vi "Keysight XSAn - Example1.vi"() -> ()   [LabVIEW 2017]
doc: "This example initializes the driver, reads a few identity interface properties, and shows a few measurements."
uses:
  <instrlib>/Keysight XSAn/Keysight XSAn.lvlib
panel:
  out "Display Details":string
  in  "DEMO POWER SUITE MEASUREMENT":T1={"Center Frequency"=50000000.0, "Input Amplitude Reference"=0, "Frequency Span"=50000000.0, "Continuous MM"=TRUE, "Scale"=10.0} {"Frequency Span" format="%#.6f"; "Center Frequency" format="%#.6f"}
  in  "DEMO TRACE DATA READ":T1={"Center Frequency"=50000000.0, "Input Amplitude Reference"=0, "Frequency Span"=50000000.0, "Continuous MM"=TRUE, "Scale"=10.0} {"Frequency Span" format="%#.6f"; "Center Frequency" format="%#.6f"}
  in  "DEMO MARKER MEASUREMENT":T2={"Center Frequency"=50000000.0, "Input Amplitude Reference"=0, "Frequency Span"=50000000.0, "Continuous MM"=TRUE} {"Frequency Span" format="%#.6f"; "Center Frequency" format="%#.6f"}
  out "RetVal":dbl[](array[numeric]) caption="Power Suit Data" format="%.2p"
  out "RetValActualSize":i32 caption="Actual Size"
  in  "RetValBufferSize":i32=100 caption="Length"
  in  "MaxTime":i32=40000 caption="Maximum Time (ms)"
  in  "RepCapIdentifier":string="PST_Results" caption="RepCapIdentifier (PST_Results)"
  out "actual points":i32 caption="Actual Points"
  out "tracedata":dbl[](array[numeric]) caption="Trace Data"
  in  "array length":i32=10 caption="Array Length"
  in  "maximum time":i32=10000 caption="Maximum Time (ms)"
  in  "trace name":string="Trace1" caption="Trace Name (Trace1)"
  in  "Trigger Source":i32=3
  in  "Span 3":dbl=-90.0 caption="Peak Threshold (dB)" format="%#.6f"
  out "Marker Amplitude":dbl caption="Marker Amplitude (dB)"
  in  "marker search (Highest)":i32(ring)=1 items=["Highest"=1, "Minimum"=2, "Next Peak"=3, "Next Peak Left"=4, "Next Peak Right"=5]
  out "Marker Frequency":dbl caption="Marker Frequency (Hz)"
  out "Simulate":bool
  out "Info":T3
  in  "Simulate":bool=TRUE
  in  "Select ?":bool=TRUE
  in  "Resource String":string="PXI0::17-0.0::INSTR"
  in  "Options String":string="DriverSetup= Model=, Trace=false, TraceName=c:\\\\temp\\\\traceOut"
  # "Keysight XSAn - Example1"
  # "------------------------------------------------------------------------------------------------------------------------------------------------------------------------------------------------------------------------"
  # "------------------------------------------------------------------------------------------------------------------------------------------------------------------------------------------------------------------------------"
  # "© Keysight Technologies  2015-2018"
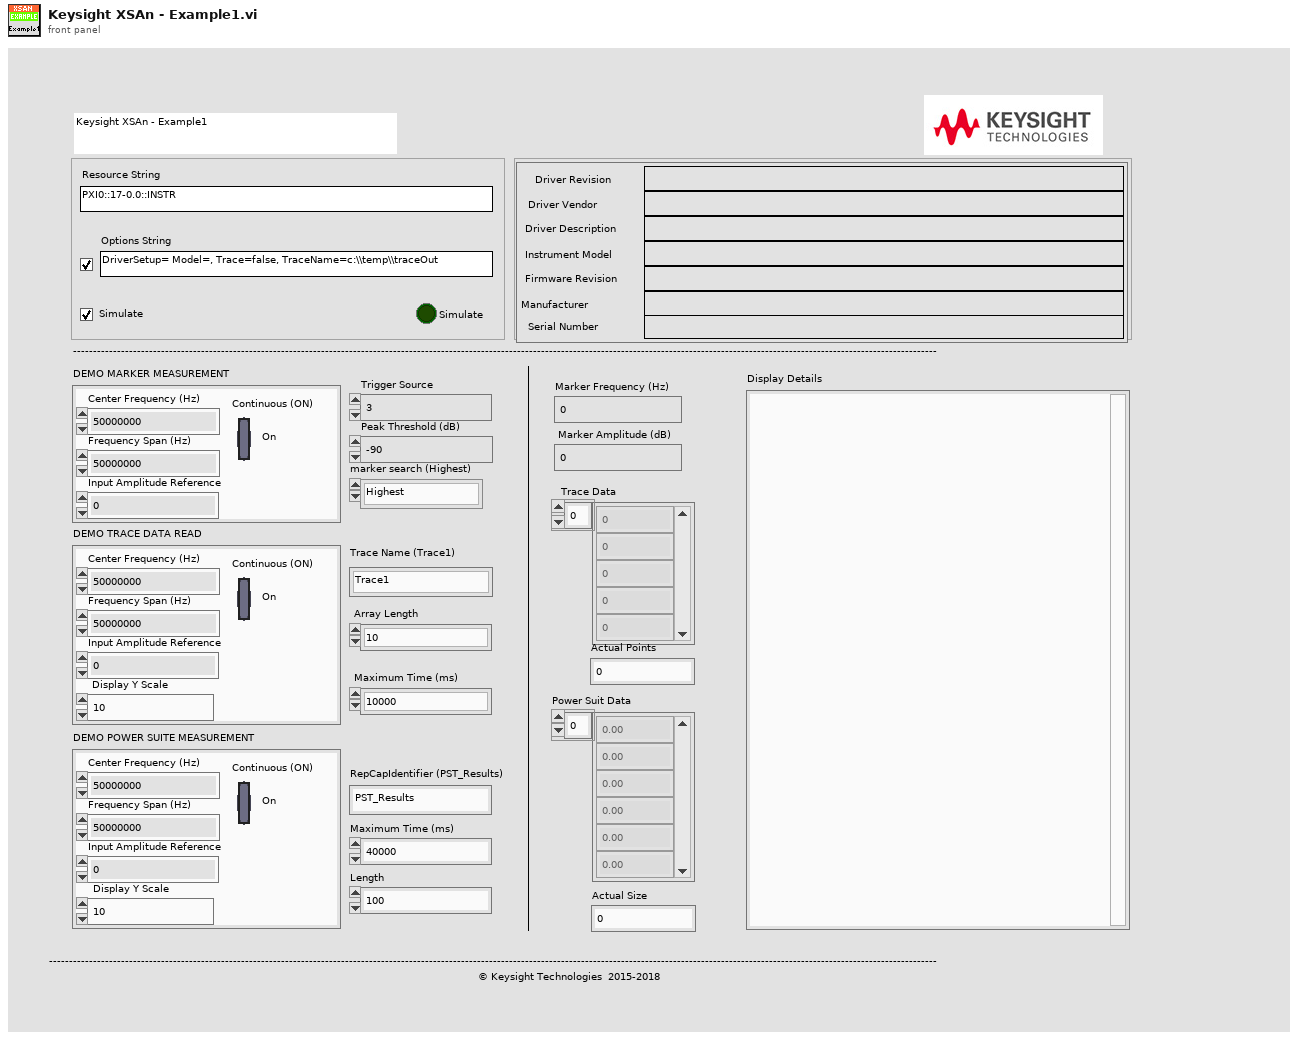
[diagram p1: front panel]
types:
  T1 = cluster{"Center Frequency":dbl, "Input Amplitude Reference":i32, "Frequency Span":dbl, "Continuous MM":bool, "Scale":dbl}
  T2 = cluster{"Center Frequency":dbl, "Input Amplitude Reference":i32, "Frequency Span":dbl, "Continuous MM":bool}
  T3 = cluster{"Driver Revision":string, "Driver Vendor":string, "Driver Description":string, "Instrument Model":string, "Firmware Revision":string, "Instrument Model 2":string, "Firmware Revision 2":string}
  T4 = cluster{"[0]":string, "[1]":string, "[2]":string, "[3]":string, "[4]":string, "[5]":string, "[6]":string}
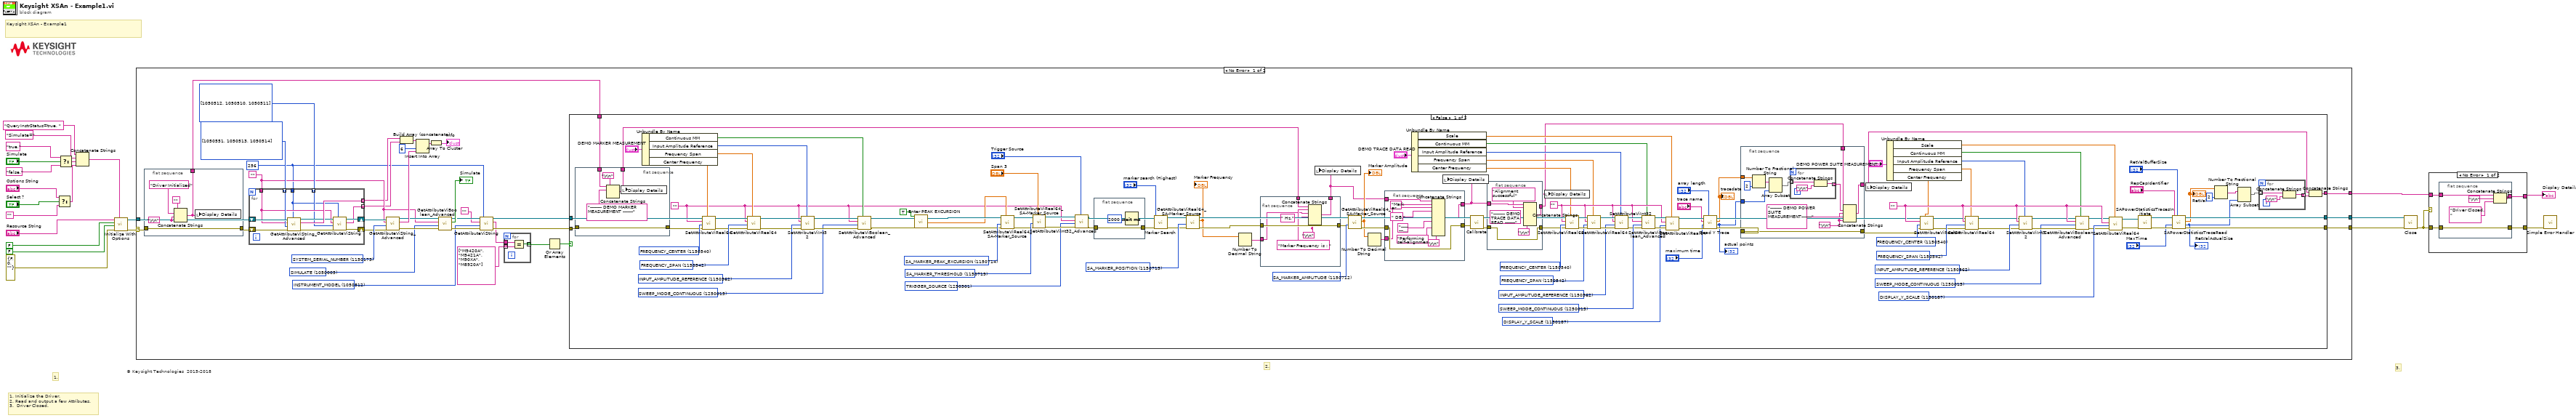
[diagram p0: block diagram]
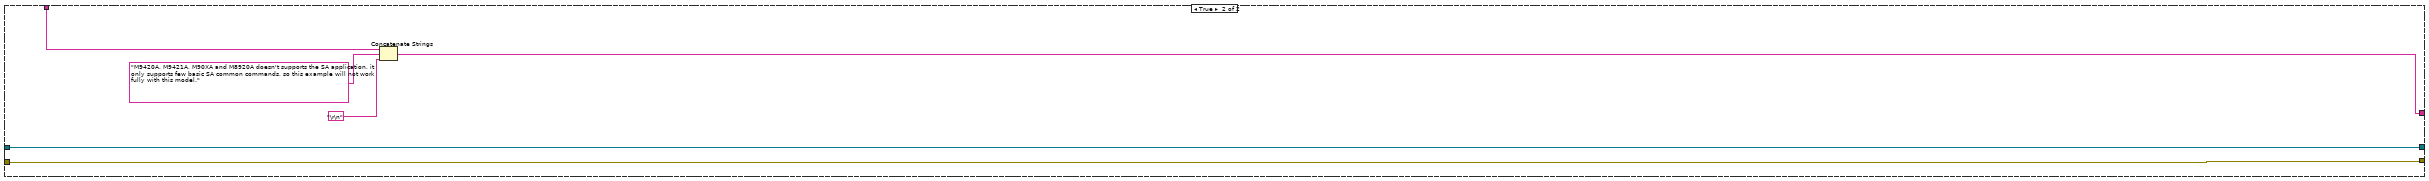
[diagram p3: hidden frame]
diagram:
  # "3."
  # "2."
  # "1."
  # "1. Initialize the Driver.\n2. Read and output a few Attributes.\n3.  Driver Closed."
  # "© Keysight Technologies  2015-2018"
  # "Keysight XSAn - Example1"
  n1 = Select(t="Options String", s="Select ?", f="") -> (s? t:f=w20:string)
  n2 = Select(t="true,", s="Simulate", f="false,") -> (s? t:f=w22:string)
  n3 = Concatenate Strings("QueryInstrStatus=true, " ("string"), "Simulate=" ("string"), w22, w20) -> (w12:string)
  n4 = call <instrlib>:"Initialize With Options.vi"("option string"=w12, "error in (no error)"=errorcluster {"status"=FALSE, "code"=0, "source"=""}, "reset device (Off)"=FALSE, "id query (Off)"=FALSE, "resource string"="Resource String") -> ("error out"=w13:errorcluster, "instrument handle out"=w7:refnum<k15>)  [unwired: 5 in]
  n5 = case shown="No Error" w13 {
    selector: w13 -> [w39 w258]
    tunnel: [w44 w258] -> w8
    tunnel: w7 -> [w37 w257]
    tunnel: [w43 w257] -> w5
    tunnel: [w35 _] -> w3
    frame No Error {
      w29 = u32 1050512 items=["ACTIVE_MARKER"=1250201, "CATALOG_CURRENT_MEASUREMENT_NAME"=1150676, "CATALOG_CURRENT_PERSONALITY_NAME"=1150677, "DISPLAY_TEXT"=1150119, "DRIVER_SETUP"=1050007, "INPUT_RF_CORRECTION_COMMENT"=1150737, "INPUT_RF_CORRECTION_DESCRIPTION"=1150738, "INSTRUMENT_FIRMWARE_REVISION"=1050510, "INSTRUMENT_MANUFACTURER"=1050511, "INSTRUMENT_MODEL"=1050512, "IO_RESOURCE_DESCRIPTOR"=1050304] ("AttributeID")
      w47 = u32 1050005 items=["IVILXISYNC_ARM_ALARM_ENABLED"=1950002, "IVILXISYNC_ARM_SOURCE_ENABLED"=1950011, "IVILXISYNC_ARM_SOURCE_OR_ENABLED"=1950014, "IVILXISYNC_EVENT_LOG_ENABLED"=1950034, "IVILXISYNC_IS_TIME_MASTER"=1950036, "IVILXISYNC_IS_TIME_SYNCHRONIZED"=1950037, "IVILXISYNC_TRIGGER_ALARM_ENABLED"=1950016, "LEVEL_ELECTRONIC_ATTENUATION_ENABLED"=1150583, "MARKER_ENABLED"=1250204, "MARKER_FREQUENCY_COUNTER_ENABLED"=1250205, "OUTPUT_ANALOG_AUTO_TYPE_ENABLED"=1150680, "PRESELECTOR_MW_ENABLED"=1150586, "RESOLUTION_BANDWIDTH_AUTO"=1250014, "SIGNAL_TRACK_ENABLED"=1250211, "SIMULATE"=1050005, "STATETRIGGER_ENABLED"=1150160, "SWEEP_MODE_CONTINUOUS"=1250015, "SWEEP_TIME_AUTO"=1250017, "SWEEP_TIME_ENABLED"=1150747, "SYSTEM_TRACE_ENABLED"=1150176, "TRACE_DISPLAY_ENABLED"=1150758, "TRACE_UPDATE_ENABLED"=1150757, "TRACES_AVERAGE_ENABLED"=1150756, "TRACES_AVERAGE_TYPE_AUTO_ENABLED"=1150667, "VIDEO_BANDWIDTH_AUTO"=1250023] ("AttributeID")
      w54 = u32 1150173 items=["IVILXISYNC_ARM_SOURCE_EVENTID"=1950012, "IVILXISYNC_ARM_SOURCE_FILTER"=1950013, "IVILXISYNC_EVENT_DESTINATION_PATH"=1950029, "IVILXISYNC_EVENT_SOURCE"=1950032, "IVILXISYNC_TRIGGER_SOURCE"=1950022, "IVILXISYNC_TRIGGER_SOURCE_EVENTID"=1950026, "IVILXISYNC_TRIGGER_SOURCE_FILTER"=1950027, "LOGICAL_NAME"=1050305, "MARKER_TRACE"=1250209, "SPECIFIC_DRIVER_DESCRIPTION"=1050514, "SPECIFIC_DRIVER_REVISION"=1050551, "SPECIFIC_DRIVER_VENDOR"=1050513, "STATETRIGGER_EVENT_ID"=1150161, "STATETRIGGER_FILTER"=1150162, "STATETRIGGER_STATE_LOCATION"=1150163, "SUPPORTED_INSTRUMENT_MODELS"=1050327, "SYSTEM_DATE"=1150172, "SYSTEM_SERIAL_NUMBER"=1150173, "SYSTEM_TIME"=1150174, "TEXT"=1150431] ("AttributeID")
      w57 = u32[] [1050512, 1050510, 1050511] items=["ACTIVE_MARKER"=1250201, "CATALOG_CURRENT_MEASUREMENT_NAME"=1150676, "CATALOG_CURRENT_PERSONALITY_NAME"=1150677, "DISPLAY_TEXT"=1150119, "DRIVER_SETUP"=1050007, "INPUT_RF_CORRECTION_COMMENT"=1150737, "INPUT_RF_CORRECTION_DESCRIPTION"=1150738, "INSTRUMENT_FIRMWARE_REVISION"=1050510, "INSTRUMENT_MANUFACTURER"=1050511, "INSTRUMENT_MODEL"=1050512, "IO_RESOURCE_DESCRIPTOR"=1050304]
      w46 = ""
      w28 = 256 ("AttributeValueBufferSize")
      w58 = u32[] [1050551, 1050513, 1050514] items=["IVILXISYNC_ARM_SOURCE_EVENTID"=1950012, "IVILXISYNC_ARM_SOURCE_FILTER"=1950013, "IVILXISYNC_EVENT_DESTINATION_PATH"=1950029, "IVILXISYNC_EVENT_SOURCE"=1950032, "IVILXISYNC_TRIGGER_SOURCE"=1950022, "IVILXISYNC_TRIGGER_SOURCE_EVENTID"=1950026, "IVILXISYNC_TRIGGER_SOURCE_FILTER"=1950027, "LOGICAL_NAME"=1050305, "MARKER_TRACE"=1250209, "SPECIFIC_DRIVER_DESCRIPTION"=1050514, "SPECIFIC_DRIVER_REVISION"=1050551, "SPECIFIC_DRIVER_VENDOR"=1050513, "STATETRIGGER_EVENT_ID"=1150161, "STATETRIGGER_FILTER"=1150162, "STATETRIGGER_STATE_LOCATION"=1150163, "SUPPORTED_INSTRUMENT_MODELS"=1050327, "SYSTEM_DATE"=1150172, "SYSTEM_SERIAL_NUMBER"=1150173, "SYSTEM_TIME"=1150174, "TEXT"=1150431]
      n6 = flat-sequence {
        tunnel: w39 -> [w66]
        tunnel: [w66] -> w38
        tunnel: [w63] -> w36
        frame #0 {
          w62 = "\r\n"
          n7 = Concatenate Strings("", "Driver Initialized", w62, w62) -> (w63:string)
          n8 = local write "Display Details"(w63) -> ()
        }
      }
      n9 = for {
        tunnel: w58 -> [w253] mode=indexing
        tunnel: [w254] -> w42 mode=indexing
        tunnel: w28 -> [w246]
        shift-right: [w250] -> w53
        shift-left: w37 -> [w256]
        shift-right: [w251] -> w52
        shift-left: w38 -> [w255]
        tunnel: w46 -> [w248]
        tunnel: w57 -> [w247] mode=indexing
        tunnel: [w245] -> w41 mode=indexing
        n10 = call <instrlib>:"GetAttributeViString_Advanced.vi"("AttributeValueBufferSize"=w246, "error in (no error)"=w255, "AttributeID"=w253, "RepCapIdentifier"=w248, "instrument handle"=w256) -> ("error out"=w252:errorcluster, "AttributeValue"=w254:string, "instrument handle out"=w249:refnum<k15>)  [unwired: 4 in]
        n11 = call <instrlib>:"GetAttributeViString.vi"("AttributeValueBufferSize"=w246, "error in (no error)"=w252, "AttributeID"=w247, "RepCapIdentifier"=w248, "instrument handle"=w249) -> ("error out"=w251:errorcluster, "AttributeValue"=w245:string, "instrument handle out"=w250:refnum<k15>)  [unwired: 4 in]
      }
      n12 = call <instrlib>:"GetAttributeViString_Advanced.vi"("error in (no error)"=w52, "AttributeID"=w54, "RepCapIdentifier"=w46, "instrument handle"=w53) -> ("error out"=w48:errorcluster, "AttributeValue"=w51:string, "instrument handle out"=w49:refnum<k15>)  [unwired: 5 in]
      n13 = Build Array (concatenate)(w42, w41) -> (w40:string[])
      n14 = Insert Into Array(array=w40, index=6, new element=w51) -> (w50:string[])
      n15 = Array To Cluster(array=w50) -> (cluster=→"Info":T4)
      n16 = call <instrlib>:"GetAttributeViBoolean_Advanced.vi"("error in (no error)"=w48, "AttributeID"=w47, "RepCapIdentifier"=w46, "instrument handle"=w49) -> ("error out"=w33:errorcluster, "AttributeValue"=→"Simulate":bool, "instrument handle out"=w34:refnum<k15>)  [unwired: 5 in]
      n17 = call <instrlib>:"GetAttributeViString.vi"("AttributeValueBufferSize"=w28, "error in (no error)"=w33, "AttributeID"=w29, "RepCapIdentifier"="", "instrument handle"=w34) -> ("error out"=w31:errorcluster, "AttributeValue"=w27:string, "instrument handle out"=w32:refnum<k15>)  [unwired: 4 in]
      n18 = for {
        tunnel: w27 -> [w61]
        tunnel: [w60] -> w25 mode=indexing
        tunnel: string[] ["M9420A", "M9421A", "M90XA", "M8920A"] -> [w59] mode=indexing
        n19 = Equal?(x=w61, y=w59) -> (x = y?=w60:bool)
      }
      n20 = Or Array Elements(Boolean array=w25) -> (logical OR=w24:bool)
      n21 = case shown="False" w24 {
        tunnel: w32 -> [w185 w244]
        tunnel: [w123 w243] -> w44
        tunnel: [w119 w244] -> w43
        tunnel: w31 -> [w97 w243]
        tunnel: w36 -> [w95 w241]
        tunnel: [w71 w239] -> w35
        frame False {
          w140 = u32 1150187 items=["ANALOGDEMODULATOR_CHANNEL_BANDWIDTH"=1150557, "ANALOGDEMODULATOR_TIME"=1150559, "ATTENUATION"=1250002, "DISPLAY_LINE"=1150191, "DISPLAY_NORMALIZED_REFERENCE"=1150184, "DISPLAY_REFERENCE_OFFSET"=1150186, "DISPLAY_REFERENCE"=1150185, "DISPLAY_Y_SCALE"=1150187, "EXTERNAL_MIXER_AVERAGE_CONVERSION_LOSS"=1250901, "EXTERNAL_MIXER_BIAS_LIMIT"=1250904, "EXTERNAL_MIXER_BIAS"=1250902, "EXTERNAL_TRIGGER_LEVEL"=1250401, "FREQUENCY_CENTER_STEP_INCREMENT"=1150541, "FREQUENCY_CENTER"=1150540, "FREQUENCY_OFFSET"=1250008, "FREQUENCY_SPAN_TO_RESOLUTION_BANDWIDTH_RATIO"=1150552, "FREQUENCY_SPAN"=1150542, "FREQUENCY_START"=1250006, "FREQUENCY_STOP"=1250007, "INPUT_IMPEDANCE"=1250009, "INPUT_RF_CENTER_FREQUENCY"=1150744, "INPUT_RF_CORRECTIONS_BASE_STATION_GAIN"=1150673, "INPUT_RF_CORRECTIONS_EXTERNAL_GAIN"=1150570, "INPUT_RF_CORRECTIONS_MOBILE_STATION_GAIN"=1150740, "INPUT_RF_MAX_MIXER_LEVEL"=1150572] ("AttributeID")
          w128 = u32 1250015 items=["IVILXISYNC_ARM_ALARM_ENABLED"=1950002, "IVILXISYNC_ARM_SOURCE_ENABLED"=1950011, "IVILXISYNC_ARM_SOURCE_OR_ENABLED"=1950014, "IVILXISYNC_EVENT_LOG_ENABLED"=1950034, "IVILXISYNC_TRIGGER_ALARM_ENABLED"=1950016, "LEVEL_ELECTRONIC_ATTENUATION_ENABLED"=1150583, "MARKER_ENABLED"=1250204, "MARKER_FREQUENCY_COUNTER_ENABLED"=1250205, "OUTPUT_ANALOG_AUTO_TYPE_ENABLED"=1150680, "PRESELECTOR_MW_ENABLED"=1150586, "RESOLUTION_BANDWIDTH_AUTO"=1250014, "SIGNAL_TRACK_ENABLED"=1250211, "SIMULATE"=1050005, "STATETRIGGER_ENABLED"=1150160, "SWEEP_MODE_CONTINUOUS"=1250015, "SWEEP_TIME_AUTO"=1250017, "SWEEP_TIME_ENABLED"=1150747, "SYSTEM_TRACE_ENABLED"=1150176, "TRACE_DISPLAY_ENABLED"=1150758, "TRACE_UPDATE_ENABLED"=1150757, "TRACES_AVERAGE_ENABLED"=1150756, "TRACES_AVERAGE_TYPE_AUTO_ENABLED"=1150667, "VIDEO_BANDWIDTH_AUTO"=1250023] ("AttributeID")
          w134 = u32 1150542 items=["ANALOGDEMODULATOR_CHANNEL_BANDWIDTH"=1150557, "ANALOGDEMODULATOR_TIME"=1150559, "ATTENUATION"=1250002, "DISPLAY_LINE"=1150191, "DISPLAY_NORMALIZED_REFERENCE"=1150184, "DISPLAY_REFERENCE_OFFSET"=1150186, "DISPLAY_REFERENCE"=1150185, "DISPLAY_Y_SCALE"=1150187, "EXTERNAL_MIXER_AVERAGE_CONVERSION_LOSS"=1250901, "EXTERNAL_MIXER_BIAS_LIMIT"=1250904, "EXTERNAL_MIXER_BIAS"=1250902, "EXTERNAL_TRIGGER_LEVEL"=1250401, "FREQUENCY_CENTER_STEP_INCREMENT"=1150541, "FREQUENCY_CENTER"=1150540, "FREQUENCY_OFFSET"=1250008, "FREQUENCY_SPAN_TO_RESOLUTION_BANDWIDTH_RATIO"=1150552, "FREQUENCY_SPAN"=1150542, "FREQUENCY_START"=1250006, "FREQUENCY_STOP"=1250007, "INPUT_IMPEDANCE"=1250009, "INPUT_RF_CENTER_FREQUENCY"=1150744, "INPUT_RF_CORRECTIONS_BASE_STATION_GAIN"=1150673, "INPUT_RF_CORRECTIONS_EXTERNAL_GAIN"=1150570, "INPUT_RF_CORRECTIONS_MOBILE_STATION_GAIN"=1150740, "INPUT_RF_MAX_MIXER_LEVEL"=1150572] ("AttributeID")
          w137 = u32 1150562 items=["AMPLITUDE_UNITS"=1250001, "ANALOGDEMODULATOR_FM_DE_EMPHASIS"=1150560, "ANALOGDEMODULATOR_TYPE"=1150556, "CALIBRATION_AUTO_ALERT_MODE"=1150674, "CALIBRATION_AUTO_ENABLED"=1150675, "DETECTOR_TYPE"=1250004, "DISPLAY_NORMALIZED_POSITION"=1150188, "DISPLAY_OPERATION_PRIORITY"=1150742, "DISPLAY_THEME"=1150155, "DISPLAY_VIEW"=1150743, "DISPLAY_WINDOW"=1150181, "EXTERNAL_MIXER_HARMONIC"=1250907, "EXTERNAL_MIXER_NUMBER_OF_PORTS"=1250908, "EXTERNAL_TRIGGER_SLOPE"=1250402, "FREQUENCY_SYNTHESIS"=1150543, "INPUT_AMPLITUDE_REFERENCE"=1150562, "INPUT_IF_FFT_IF_GAIN_STATE"=1150565, "INPUT_IF_SWEPT_IF_GAIN_STATE"=1150568, "INPUT_PORT"=1150563, "INPUT_RF_CORRECTION_ANTENNA_UNIT"=1150736, "INPUT_RF_CORRECTION_FREQUENCY_INTERPOLATION"=1150575, "INPUT_RF_CORRECTIONS_IMPEDANCE"=1150739, "INPUT_RF_COUPLING"=1150571, "INPUT_TYPE"=1150774] ("AttributeID")
          w141 = ""
          w136 = u32 1150540 items=["ANALOGDEMODULATOR_CHANNEL_BANDWIDTH"=1150557, "ANALOGDEMODULATOR_TIME"=1150559, "ATTENUATION"=1250002, "DISPLAY_LINE"=1150191, "DISPLAY_NORMALIZED_REFERENCE"=1150184, "DISPLAY_REFERENCE_OFFSET"=1150186, "DISPLAY_REFERENCE"=1150185, "DISPLAY_Y_SCALE"=1150187, "EXTERNAL_MIXER_AVERAGE_CONVERSION_LOSS"=1250901, "EXTERNAL_MIXER_BIAS_LIMIT"=1250904, "EXTERNAL_MIXER_BIAS"=1250902, "EXTERNAL_TRIGGER_LEVEL"=1250401, "FREQUENCY_CENTER_STEP_INCREMENT"=1150541, "FREQUENCY_CENTER"=1150540, "FREQUENCY_OFFSET"=1250008, "FREQUENCY_SPAN_TO_RESOLUTION_BANDWIDTH_RATIO"=1150552, "FREQUENCY_SPAN"=1150542, "FREQUENCY_START"=1250006, "FREQUENCY_STOP"=1250007, "INPUT_IMPEDANCE"=1250009, "INPUT_RF_CENTER_FREQUENCY"=1150744, "INPUT_RF_CORRECTIONS_BASE_STATION_GAIN"=1150673, "INPUT_RF_CORRECTIONS_EXTERNAL_GAIN"=1150570, "INPUT_RF_CORRECTIONS_MOBILE_STATION_GAIN"=1150740, "INPUT_RF_MAX_MIXER_LEVEL"=1150572] ("AttributeID")
          w148 = u32 1250301 items=["IVILXISYNC_ARM_ALARM_COUNT"=1950001, "IVILXISYNC_ARM_ALARM_REPEAT_COUNT"=1950004, "IVILXISYNC_ARM_COUNT"=1950007, "IVILXISYNC_ARM_SOURCE_COUNT"=1950009, "IVILXISYNC_ARM_SOURCE_DETECTION"=1950010, "IVILXISYNC_EVENT_COUNT"=1950028, "IVILXISYNC_EVENT_DRIVE_MODE"=1950030, "IVILXISYNC_EVENT_LOG_ENTRY_COUNT"=1950035, "IVILXISYNC_EVENT_SLOPE"=1950031, "IVILXISYNC_EVENT_WIRED_OR_BIAS_MODE"=1950033, "IVILXISYNC_TRIGGER_ALARM_COUNT"=1950015, "IVILXISYNC_TRIGGER_ALARM_REPEAT_COUNT"=1950018, "IVILXISYNC_TRIGGER_COUNT"=1950021, "IVILXISYNC_TRIGGER_SOURCE_COUNT"=1950023, "IVILXISYNC_TRIGGER_SOURCE_DETECTION"=1950025, "LEVEL_ATTENUATION_OPTIMIZE"=1150012, "LEVEL_ATTENUATION_STEP_INCREMENT"=1150013, "LEVEL_ELECTRONIC_ATTENUATION"=1150578, "MARKER_COUNT"=1250203, "MARKER_TYPE"=1250701, "MEMORYOPERATION_SCREEN_IMAGE_THEME"=1150678, "NUMBER_OF_DIVISIONS"=1250602, "NUMBER_OF_SWEEPS"=1250010, "OUTPUT_ANALOG_TYPE"=1150679, "OUTPUT_AUXILIARY_IF_TYPE"=1150681, "PRESELECTOR_MW_PATH"=1150585, "RADIO_BAND_CLASS"=1150550, "RADIO_DEVICE"=1150547, "RADIO_NON_STANDARD_MEASUREMENT_ENABLED"=1150549, "RADIO_PACKET_TYPE"=1150551, "RADIO_STANDARD"=1150548, "REFOSCILLATOR_EXTERNAL_BANDWIDTH"=1150539, "REFOSCILLATOR_EXTERNAL_COUPLING"=1150538, "STATETRIGGER_DETECTION"=1150159, "STATUS_SERIAL_POLL"=1150759, "SYSTEM_IO_TIMEOUT"=1150783, "SYSTEM_TIMEOUT_MILLISECONDS"=1150175, "TRACE_COUNT"=1250018, "TRACE_DETECTOR_TYPE"=1150782, "TRACE_SIZE"=1250019, "TRACE_TYPE"=1250020, "TRACES_AVERAGE_TYPE"=1150666, "TRIGGER_EXTERNAL2_SLOPE"=1150671, "TRIGGER_SOURCE"=1250301, "VERTICAL_SCALE"=1250021, "VIDEO_TRIGGER_SLOPE"=1250502] ("AttributeID")
          w156 = u32 1150719 items=["SA_MARKER_FREQUENCYCOUNTER_GATE_TIME"=1150683, "SA_MARKER_FUNCTION_BAND_LEFT"=1150693, "SA_MARKER_FUNCTION_BAND_RIGHT"=1150694, "SA_MARKER_FUNCTION_BAND_SPAN"=1150695, "SA_MARKER_NDBPOINTS_VALUE"=1150687, "SA_MARKER_PEAK_EXCURSION"=1150714, "SA_MARKER_POSITION"=1150715, "SA_MARKER_THRESHOLD"=1150719, "SA_MARKER_X_AXIS_TRACE_POINTS"=1150710, "SA_MARKER_Y"=1150702, "SA_SOURCE_FREQUENCY_OFFSET"=1150797, "SA_SOURCE_LEVEL_AMPLITUDE"=1150785, "SA_SOURCE_LEVEL_AMPLITUDE_OFFSET"=1150790, "SA_SOURCE_LEVEL_AMPLITUDE_STEP"=1150791, "SA_SOURCE_LEVEL_POWER_SWEEP"=1150788, "SA_SOURCE_LEVEL_TRACK_DELAY"=1150793] ("AttributeID")
          w157 = u32 1150714 items=["SA_MARKER_FREQUENCYCOUNTER_GATE_TIME"=1150683, "SA_MARKER_FUNCTION_BAND_LEFT"=1150693, "SA_MARKER_FUNCTION_BAND_RIGHT"=1150694, "SA_MARKER_FUNCTION_BAND_SPAN"=1150695, "SA_MARKER_NDBPOINTS_VALUE"=1150687, "SA_MARKER_PEAK_EXCURSION"=1150714, "SA_MARKER_POSITION"=1150715, "SA_MARKER_THRESHOLD"=1150719, "SA_MARKER_X_AXIS_TRACE_POINTS"=1150710, "SA_MARKER_Y"=1150702, "SA_SOURCE_FREQUENCY_OFFSET"=1150797, "SA_SOURCE_LEVEL_AMPLITUDE"=1150785, "SA_SOURCE_LEVEL_AMPLITUDE_OFFSET"=1150790, "SA_SOURCE_LEVEL_AMPLITUDE_STEP"=1150791, "SA_SOURCE_LEVEL_POWER_SWEEP"=1150788, "SA_SOURCE_LEVEL_TRACK_DELAY"=1150793] ("AttributeID")
          w160 = u32 1150187 items=["ANALOGDEMODULATOR_CHANNEL_BANDWIDTH"=1150557, "ANALOGDEMODULATOR_TIME"=1150559, "ATTENUATION"=1250002, "DISPLAY_LINE"=1150191, "DISPLAY_NORMALIZED_REFERENCE"=1150184, "DISPLAY_REFERENCE_OFFSET"=1150186, "DISPLAY_REFERENCE"=1150185, "DISPLAY_Y_SCALE"=1150187, "EXTERNAL_MIXER_AVERAGE_CONVERSION_LOSS"=1250901, "EXTERNAL_MIXER_BIAS_LIMIT"=1250904, "EXTERNAL_MIXER_BIAS"=1250902, "EXTERNAL_TRIGGER_LEVEL"=1250401, "FREQUENCY_CENTER_STEP_INCREMENT"=1150541, "FREQUENCY_CENTER"=1150540, "FREQUENCY_OFFSET"=1250008, "FREQUENCY_SPAN_TO_RESOLUTION_BANDWIDTH_RATIO"=1150552, "FREQUENCY_SPAN"=1150542, "FREQUENCY_START"=1250006, "FREQUENCY_STOP"=1250007, "INPUT_IMPEDANCE"=1250009, "INPUT_RF_CENTER_FREQUENCY"=1150744, "INPUT_RF_CORRECTIONS_BASE_STATION_GAIN"=1150673, "INPUT_RF_CORRECTIONS_EXTERNAL_GAIN"=1150570, "INPUT_RF_CORRECTIONS_MOBILE_STATION_GAIN"=1150740, "INPUT_RF_MAX_MIXER_LEVEL"=1150572] ("AttributeID")
          w173 = u32 1250015 items=["IVILXISYNC_ARM_ALARM_ENABLED"=1950002, "IVILXISYNC_ARM_SOURCE_ENABLED"=1950011, "IVILXISYNC_ARM_SOURCE_OR_ENABLED"=1950014, "IVILXISYNC_EVENT_LOG_ENABLED"=1950034, "IVILXISYNC_TRIGGER_ALARM_ENABLED"=1950016, "LEVEL_ELECTRONIC_ATTENUATION_ENABLED"=1150583, "MARKER_ENABLED"=1250204, "MARKER_FREQUENCY_COUNTER_ENABLED"=1250205, "OUTPUT_ANALOG_AUTO_TYPE_ENABLED"=1150680, "PRESELECTOR_MW_ENABLED"=1150586, "RESOLUTION_BANDWIDTH_AUTO"=1250014, "SIGNAL_TRACK_ENABLED"=1250211, "SIMULATE"=1050005, "STATETRIGGER_ENABLED"=1150160, "SWEEP_MODE_CONTINUOUS"=1250015, "SWEEP_TIME_AUTO"=1250017, "SWEEP_TIME_ENABLED"=1150747, "SYSTEM_TRACE_ENABLED"=1150176, "TRACE_DISPLAY_ENABLED"=1150758, "TRACE_UPDATE_ENABLED"=1150757, "TRACES_AVERAGE_ENABLED"=1150756, "TRACES_AVERAGE_TYPE_AUTO_ENABLED"=1150667, "VIDEO_BANDWIDTH_AUTO"=1250023] ("AttributeID")
          w167 = u32 1150542 items=["ANALOGDEMODULATOR_CHANNEL_BANDWIDTH"=1150557, "ANALOGDEMODULATOR_TIME"=1150559, "ATTENUATION"=1250002, "DISPLAY_LINE"=1150191, "DISPLAY_NORMALIZED_REFERENCE"=1150184, "DISPLAY_REFERENCE_OFFSET"=1150186, "DISPLAY_REFERENCE"=1150185, "DISPLAY_Y_SCALE"=1150187, "EXTERNAL_MIXER_AVERAGE_CONVERSION_LOSS"=1250901, "EXTERNAL_MIXER_BIAS_LIMIT"=1250904, "EXTERNAL_MIXER_BIAS"=1250902, "EXTERNAL_TRIGGER_LEVEL"=1250401, "FREQUENCY_CENTER_STEP_INCREMENT"=1150541, "FREQUENCY_CENTER"=1150540, "FREQUENCY_OFFSET"=1250008, "FREQUENCY_SPAN_TO_RESOLUTION_BANDWIDTH_RATIO"=1150552, "FREQUENCY_SPAN"=1150542, "FREQUENCY_START"=1250006, "FREQUENCY_STOP"=1250007, "INPUT_IMPEDANCE"=1250009, "INPUT_RF_CENTER_FREQUENCY"=1150744, "INPUT_RF_CORRECTIONS_BASE_STATION_GAIN"=1150673, "INPUT_RF_CORRECTIONS_EXTERNAL_GAIN"=1150570, "INPUT_RF_CORRECTIONS_MOBILE_STATION_GAIN"=1150740, "INPUT_RF_MAX_MIXER_LEVEL"=1150572] ("AttributeID")
          w164 = u32 1150562 items=["AMPLITUDE_UNITS"=1250001, "ANALOGDEMODULATOR_FM_DE_EMPHASIS"=1150560, "ANALOGDEMODULATOR_TYPE"=1150556, "CALIBRATION_AUTO_ALERT_MODE"=1150674, "CALIBRATION_AUTO_ENABLED"=1150675, "DETECTOR_TYPE"=1250004, "DISPLAY_NORMALIZED_POSITION"=1150188, "DISPLAY_OPERATION_PRIORITY"=1150742, "DISPLAY_THEME"=1150155, "DISPLAY_VIEW"=1150743, "DISPLAY_WINDOW"=1150181, "EXTERNAL_MIXER_HARMONIC"=1250907, "EXTERNAL_MIXER_NUMBER_OF_PORTS"=1250908, "EXTERNAL_TRIGGER_SLOPE"=1250402, "FREQUENCY_SYNTHESIS"=1150543, "INPUT_AMPLITUDE_REFERENCE"=1150562, "INPUT_IF_FFT_IF_GAIN_STATE"=1150565, "INPUT_IF_SWEPT_IF_GAIN_STATE"=1150568, "INPUT_PORT"=1150563, "INPUT_RF_CORRECTION_ANTENNA_UNIT"=1150736, "INPUT_RF_CORRECTION_FREQUENCY_INTERPOLATION"=1150575, "INPUT_RF_CORRECTIONS_IMPEDANCE"=1150739, "INPUT_RF_COUPLING"=1150571, "INPUT_TYPE"=1150774] ("AttributeID")
          w159 = ""
          w165 = u32 1150540 items=["ANALOGDEMODULATOR_CHANNEL_BANDWIDTH"=1150557, "ANALOGDEMODULATOR_TIME"=1150559, "ATTENUATION"=1250002, "DISPLAY_LINE"=1150191, "DISPLAY_NORMALIZED_REFERENCE"=1150184, "DISPLAY_REFERENCE_OFFSET"=1150186, "DISPLAY_REFERENCE"=1150185, "DISPLAY_Y_SCALE"=1150187, "EXTERNAL_MIXER_AVERAGE_CONVERSION_LOSS"=1250901, "EXTERNAL_MIXER_BIAS_LIMIT"=1250904, "EXTERNAL_MIXER_BIAS"=1250902, "EXTERNAL_TRIGGER_LEVEL"=1250401, "FREQUENCY_CENTER_STEP_INCREMENT"=1150541, "FREQUENCY_CENTER"=1150540, "FREQUENCY_OFFSET"=1250008, "FREQUENCY_SPAN_TO_RESOLUTION_BANDWIDTH_RATIO"=1150552, "FREQUENCY_SPAN"=1150542, "FREQUENCY_START"=1250006, "FREQUENCY_STOP"=1250007, "INPUT_IMPEDANCE"=1250009, "INPUT_RF_CENTER_FREQUENCY"=1150744, "INPUT_RF_CORRECTIONS_BASE_STATION_GAIN"=1150673, "INPUT_RF_CORRECTIONS_EXTERNAL_GAIN"=1150570, "INPUT_RF_CORRECTIONS_MOBILE_STATION_GAIN"=1150740, "INPUT_RF_MAX_MIXER_LEVEL"=1150572] ("AttributeID")
          w174 = u32 1250015 items=["IVILXISYNC_ARM_ALARM_ENABLED"=1950002, "IVILXISYNC_ARM_SOURCE_ENABLED"=1950011, "IVILXISYNC_ARM_SOURCE_OR_ENABLED"=1950014, "IVILXISYNC_EVENT_LOG_ENABLED"=1950034, "IVILXISYNC_TRIGGER_ALARM_ENABLED"=1950016, "LEVEL_ELECTRONIC_ATTENUATION_ENABLED"=1150583, "MARKER_ENABLED"=1250204, "MARKER_FREQUENCY_COUNTER_ENABLED"=1250205, "OUTPUT_ANALOG_AUTO_TYPE_ENABLED"=1150680, "PRESELECTOR_MW_ENABLED"=1150586, "RESOLUTION_BANDWIDTH_AUTO"=1250014, "SIGNAL_TRACK_ENABLED"=1250211, "SIMULATE"=1050005, "STATETRIGGER_ENABLED"=1150160, "SWEEP_MODE_CONTINUOUS"=1250015, "SWEEP_TIME_AUTO"=1250017, "SWEEP_TIME_ENABLED"=1150747, "SYSTEM_TRACE_ENABLED"=1150176, "TRACE_DISPLAY_ENABLED"=1150758, "TRACE_UPDATE_ENABLED"=1150757, "TRACES_AVERAGE_ENABLED"=1150756, "TRACES_AVERAGE_TYPE_AUTO_ENABLED"=1150667, "VIDEO_BANDWIDTH_AUTO"=1250023] ("AttributeID")
          w182 = u32 1150715 items=["SA_MARKER_AMPLITUDE"=1150712, "SA_MARKER_FREQUENCYCOUNTER_GATE_TIME"=1150683, "SA_MARKER_FUNCTION_BAND_LEFT"=1150693, "SA_MARKER_FUNCTION_BAND_RIGHT"=1150694, "SA_MARKER_FUNCTION_BAND_SPAN"=1150695, "SA_MARKER_NDBPOINTS_RESULTS"=1150688, "SA_MARKER_NDBPOINTS_VALUE"=1150687, "SA_MARKER_PEAK_EXCURSION"=1150714, "SA_MARKER_POSITION"=1150715, "SA_MARKER_REFERENCE_AMPLITUDE"=1150716, "SA_MARKER_REFERENCE_POSITION"=1150717, "SA_MARKER_THRESHOLD"=1150719, "SA_MARKER_X_AXIS_TRACE_POINTS"=1150710, "SA_MARKER_Y"=1150702, "SA_SOURCE_FREQUENCY_OFFSET"=1150797, "SA_SOURCE_LEVEL_AMPLITUDE"=1150785, "SA_SOURCE_LEVEL_AMPLITUDE_OFFSET"=1150790, "SA_SOURCE_LEVEL_AMPLITUDE_STEP"=1150791, "SA_SOURCE_LEVEL_POWER_SWEEP"=1150788, "SA_SOURCE_LEVEL_TRACK_DELAY"=1150793] ("AttributeID")
          w181 = u32 1150712 items=["SA_MARKER_AMPLITUDE"=1150712, "SA_MARKER_FREQUENCYCOUNTER_GATE_TIME"=1150683, "SA_MARKER_FUNCTION_BAND_LEFT"=1150693, "SA_MARKER_FUNCTION_BAND_RIGHT"=1150694, "SA_MARKER_FUNCTION_BAND_SPAN"=1150695, "SA_MARKER_NDBPOINTS_RESULTS"=1150688, "SA_MARKER_NDBPOINTS_VALUE"=1150687, "SA_MARKER_PEAK_EXCURSION"=1150714, "SA_MARKER_POSITION"=1150715, "SA_MARKER_REFERENCE_AMPLITUDE"=1150716, "SA_MARKER_REFERENCE_POSITION"=1150717, "SA_MARKER_THRESHOLD"=1150719, "SA_MARKER_X_AXIS_TRACE_POINTS"=1150710, "SA_MARKER_Y"=1150702, "SA_SOURCE_FREQUENCY_OFFSET"=1150797, "SA_SOURCE_LEVEL_AMPLITUDE"=1150785, "SA_SOURCE_LEVEL_AMPLITUDE_OFFSET"=1150790, "SA_SOURCE_LEVEL_AMPLITUDE_STEP"=1150791, "SA_SOURCE_LEVEL_POWER_SWEEP"=1150788, "SA_SOURCE_LEVEL_TRACK_DELAY"=1150793] ("AttributeID")
          w189 = u32 1150542 items=["ANALOGDEMODULATOR_CHANNEL_BANDWIDTH"=1150557, "ANALOGDEMODULATOR_TIME"=1150559, "ATTENUATION"=1250002, "DISPLAY_LINE"=1150191, "DISPLAY_NORMALIZED_REFERENCE"=1150184, "DISPLAY_REFERENCE_OFFSET"=1150186, "DISPLAY_REFERENCE"=1150185, "DISPLAY_Y_SCALE"=1150187, "EXTERNAL_MIXER_AVERAGE_CONVERSION_LOSS"=1250901, "EXTERNAL_MIXER_BIAS_LIMIT"=1250904, "EXTERNAL_MIXER_BIAS"=1250902, "EXTERNAL_TRIGGER_LEVEL"=1250401, "FREQUENCY_CENTER_STEP_INCREMENT"=1150541, "FREQUENCY_CENTER"=1150540, "FREQUENCY_OFFSET"=1250008, "FREQUENCY_SPAN_TO_RESOLUTION_BANDWIDTH_RATIO"=1150552, "FREQUENCY_SPAN"=1150542, "FREQUENCY_START"=1250006, "FREQUENCY_STOP"=1250007, "INPUT_IMPEDANCE"=1250009, "INPUT_RF_CENTER_FREQUENCY"=1150744, "INPUT_RF_CORRECTIONS_BASE_STATION_GAIN"=1150673, "INPUT_RF_CORRECTIONS_EXTERNAL_GAIN"=1150570, "INPUT_RF_CORRECTIONS_MOBILE_STATION_GAIN"=1150740, "INPUT_RF_MAX_MIXER_LEVEL"=1150572] ("AttributeID")
          w192 = u32 1150562 items=["AMPLITUDE_UNITS"=1250001, "ANALOGDEMODULATOR_FM_DE_EMPHASIS"=1150560, "ANALOGDEMODULATOR_TYPE"=1150556, "CALIBRATION_AUTO_ALERT_MODE"=1150674, "CALIBRATION_AUTO_ENABLED"=1150675, "DETECTOR_TYPE"=1250004, "DISPLAY_NORMALIZED_POSITION"=1150188, "DISPLAY_OPERATION_PRIORITY"=1150742, "DISPLAY_THEME"=1150155, "DISPLAY_VIEW"=1150743, "DISPLAY_WINDOW"=1150181, "EXTERNAL_MIXER_HARMONIC"=1250907, "EXTERNAL_MIXER_NUMBER_OF_PORTS"=1250908, "EXTERNAL_TRIGGER_SLOPE"=1250402, "FREQUENCY_SYNTHESIS"=1150543, "INPUT_AMPLITUDE_REFERENCE"=1150562, "INPUT_IF_FFT_IF_GAIN_STATE"=1150565, "INPUT_IF_SWEPT_IF_GAIN_STATE"=1150568, "INPUT_PORT"=1150563, "INPUT_RF_CORRECTION_ANTENNA_UNIT"=1150736, "INPUT_RF_CORRECTION_FREQUENCY_INTERPOLATION"=1150575, "INPUT_RF_CORRECTIONS_IMPEDANCE"=1150739, "INPUT_RF_COUPLING"=1150571, "INPUT_TYPE"=1150774] ("AttributeID")
          w77 = ""
          w191 = u32 1150540 items=["ANALOGDEMODULATOR_CHANNEL_BANDWIDTH"=1150557, "ANALOGDEMODULATOR_TIME"=1150559, "ATTENUATION"=1250002, "DISPLAY_LINE"=1150191, "DISPLAY_NORMALIZED_REFERENCE"=1150184, "DISPLAY_REFERENCE_OFFSET"=1150186, "DISPLAY_REFERENCE"=1150185, "DISPLAY_Y_SCALE"=1150187, "EXTERNAL_MIXER_AVERAGE_CONVERSION_LOSS"=1250901, "EXTERNAL_MIXER_BIAS_LIMIT"=1250904, "EXTERNAL_MIXER_BIAS"=1250902, "EXTERNAL_TRIGGER_LEVEL"=1250401, "FREQUENCY_CENTER_STEP_INCREMENT"=1150541, "FREQUENCY_CENTER"=1150540, "FREQUENCY_OFFSET"=1250008, "FREQUENCY_SPAN_TO_RESOLUTION_BANDWIDTH_RATIO"=1150552, "FREQUENCY_SPAN"=1150542, "FREQUENCY_START"=1250006, "FREQUENCY_STOP"=1250007, "INPUT_IMPEDANCE"=1250009, "INPUT_RF_CENTER_FREQUENCY"=1150744, "INPUT_RF_CORRECTIONS_BASE_STATION_GAIN"=1150673, "INPUT_RF_CORRECTIONS_EXTERNAL_GAIN"=1150570, "INPUT_RF_CORRECTIONS_MOBILE_STATION_GAIN"=1150740, "INPUT_RF_MAX_MIXER_LEVEL"=1150572] ("AttributeID")
          n22 = flat-sequence {
            tunnel: w97 -> [w236]
            tunnel: [w236] -> w96
            tunnel: w95 -> [w235]
            tunnel: [w233] -> w92
            frame #0 {
              w232 = "\r\n"
              n23 = Concatenate Strings(w235, "-------- DEMO MARKER MEASUREMENT -------" ("y"), w232, w232) -> (w233:string)
              n24 = local write "Display Details"(w233) -> ()
            }
          }
          n25 = Unbundle By Name("DEMO MARKER MEASUREMENT") -> ("Continuous MM"=w113:bool, "Input Amplitude Reference"=w112:i32, "Frequency Span"=w111:dbl, "Center Frequency"=w110:dbl)
          n26 = call <instrlib>:"SetAttributeViReal64.vi"("AttributeValue"=w110, "error in (no error)"=w96, "AttributeID"=w191, "RepCapIdentifier"=w77, "instrument handle"=w185) -> ("error out"=w186:errorcluster, "instrument handle out"=w190:refnum<k15>)  [unwired: 5 in]
          n27 = call <instrlib>:"SetAttributeViReal64.vi"("AttributeValue"=w111, "error in (no error)"=w186, "AttributeID"=w189, "RepCapIdentifier"=w77, "instrument handle"=w190) -> ("error out"=w187:errorcluster, "instrument handle out"=w188:refnum<k15>)  [unwired: 5 in]
          n28 = call <instrlib>:"SetAttributeViInt32.vi"("AttributeValue"=w112, "error in (no error)"=w187, "AttributeID"=w192, "RepCapIdentifier"=w77, "instrument handle"=w188) -> ("error out"=w175:errorcluster, "instrument handle out"=w176:refnum<k15>)  [unwired: 5 in]
          n29 = call <instrlib>:"SetAttributeViBoolean_Advanced.vi"("AttributeValue (Off)"=w113, "error in (no error)"=w175, "AttributeID"=w174, "RepCapIdentifier"=w77, "instrument handle"=w176) -> ("error out"=w118:errorcluster, "instrument handle out"=w158:refnum<k15>)  [unwired: 5 in]
          n30 = call "Enter PEAK EXCURSION"("Enable"=TRUE, "error in (no error)"=w118) -> ("PEAK EXCURSION"=w116:dbl, "error out"=w117:errorcluster)  [unwired: 15 in, 1 out]
          n31 = call <instrlib>:"SetAttributeViReal64_SA-Marker_Source.vi"("AttributeValue"=w116, "error in (no error)"=w117, "AttributeID"=w157, "instrument handle"=w158) -> ("error out"=w154:errorcluster, "instrument handle out"=w155:refnum<k15>)  [unwired: 6 in]
          n32 = call <instrlib>:"SetAttributeViReal64_SA-Marker_Source.vi"("AttributeValue"="Span 3", "error in (no error)"=w154, "AttributeID"=w156, "instrument handle"=w155) -> ("error out"=w151:errorcluster, "instrument handle out"=w152:refnum<k15>)  [unwired: 6 in]
          n33 = call <instrlib>:"SetAttributeViInt32_Advanced.vi"("AttributeValue"="Trigger Source", "error in (no error)"=w151, "AttributeID"=w148, "RepCapIdentifier"=w77, "instrument handle"=w152) -> ("error out"=w149:errorcluster, "instrument handle out"=w150:refnum<k15>)  [unwired: 5 in]
          n34 = flat-sequence {
            tunnel: w149 -> [w237]
            tunnel: [w237] -> w184
            frame #0 {
              n35 = Wait (ms)(milliseconds to wait=u32 2000) -> ()  [unwired: 1 out]
            }
          }
          n36 = call <instrlib>:"Marker Search.vi"("error in (no error)"=w184, "marker search (Highest)"="marker search (Highest)", "instrument handle"=w150) -> ("error out"=w178:errorcluster, "instrument handle out"=w180:refnum<k15>)  [unwired: 7 in]
          n37 = call <instrlib>:"GetAttributeViReal64_SA-Marker_Source.vi"("error in (no error)"=w178, "AttributeID"=w182, "instrument handle"=w180) -> ("error out"=w94:errorcluster, "AttributeValue"=w91:dbl, "instrument handle out"=w179:refnum<k15>)  [unwired: 6 in]
          "Marker Frequency" <- w91
          n38 = Number To Decimal String(number=w91) -> (decimal integer string=w90:string)  [unwired: 1 in]
          n39 = flat-sequence {
            tunnel: w94 -> [w231]
            tunnel: [w231] -> w93
            tunnel: w92 -> [w230]
            tunnel: w90 -> [w228]
            tunnel: [w226] -> w85
            frame #0 {
              w225 = "\r\n"
              n40 = Concatenate Strings(w230, "Marker Frequency is : ", w228, " Hz.", w225, w225) -> (w226:string)
            }
          }
          n41 = local write "Display Details"(w85) -> ()
          n42 = call <instrlib>:"GetAttributeViReal64_SA-Marker_Source.vi"("error in (no error)"=w93, "AttributeID"=w181, "instrument handle"=w179) -> ("error out"=w89:errorcluster, "AttributeValue"=w87:dbl, "instrument handle out"=w177:refnum<k15>)  [unwired: 6 in]
          "Marker Amplitude" <- w87
          n43 = Number To Decimal String(number=w87) -> (decimal integer string=w86:string)  [unwired: 1 in]
          n44 = flat-sequence {
            tunnel: [w224] -> w83
            tunnel: w89 -> [w221]
            tunnel: [w221] -> w88
            tunnel: w86 -> [w220]
            tunnel: w85 -> [w219]
            frame #0 {
              w216 = "\r\n"
              n45 = Concatenate Strings(w219, "Marker Amplitude is : ", w220, " DB.", w216, w216, "-------- DEMO INTERNAL ALIGNMENT -------" ("y"), w216, "Performing self-alignment..." ("y"), w216, w216) -> (w224:string)
            }
          }
          n46 = Unbundle By Name("DEMO TRACE DATA READ") -> ("Scale"=w99:dbl, "Continuous MM"=w105:bool, "Input Amplitude Reference"=w106:i32, "Frequency Span"=w107:dbl, "Center Frequency"=w108:dbl)
          n47 = local write "Display Details"(w83) -> ()
          n48 = call <instrlib>:"Calibrate.vi"("error in (no error)"=w88, "instrument handle"=w177) -> ("error out"=w84:errorcluster, "instrument handle out"=w163:refnum<k15>)  [unwired: 8 in]
          n49 = flat-sequence {
            tunnel: w84 -> [w212]
            tunnel: w83 -> [w215]
            tunnel: [w213] -> w79
            tunnel: [w212] -> w82
            frame #0 {
              w210 = "\r\n"
              n50 = Concatenate Strings(w215, "Alignment successful" ("y"), w210, w210, "-------- DEMO TRACE DATA READ -------" ("y"), w210, w210) -> (w213:string)
            }
          }
          n51 = local write "Display Details"(w79) -> ()
          n52 = call <instrlib>:"SetAttributeViReal64.vi"("AttributeValue"=w108, "error in (no error)"=w82, "AttributeID"=w165, "RepCapIdentifier"=w159, "instrument handle"=w163) -> ("error out"=w170:errorcluster, "instrument handle out"=w166:refnum<k15>)  [unwired: 5 in]
          n53 = call <instrlib>:"SetAttributeViReal64.vi"("AttributeValue"=w107, "error in (no error)"=w170, "AttributeID"=w167, "RepCapIdentifier"=w159, "instrument handle"=w166) -> ("error out"=w169:errorcluster, "instrument handle out"=w168:refnum<k15>)  [unwired: 5 in]
          n54 = call <instrlib>:"SetAttributeViInt32.vi"("AttributeValue"=w106, "error in (no error)"=w169, "AttributeID"=w164, "RepCapIdentifier"=w159, "instrument handle"=w168) -> ("error out"=w172:errorcluster, "instrument handle out"=w171:refnum<k15>)  [unwired: 5 in]
          n55 = call <instrlib>:"SetAttributeViBoolean_Advanced.vi"("AttributeValue (Off)"=w105, "error in (no error)"=w172, "AttributeID"=w173, "RepCapIdentifier"=w159, "instrument handle"=w171) -> ("error out"=w161:errorcluster, "instrument handle out"=w162:refnum<k15>)  [unwired: 5 in]
          n56 = call <instrlib>:"SetAttributeViReal64.vi"("AttributeValue"=w99, "error in (no error)"=w161, "AttributeID"=w160, "RepCapIdentifier"=w159, "instrument handle"=w162) -> ("error out"=w145:errorcluster, "instrument handle out"=w146:refnum<k15>)  [unwired: 5 in]
          n57 = call <instrlib>:"Read Y Trace.vi"("array length"="array length", "error in (no error)"=w145, "maximum time"="maximum time", "trace name"="trace name", "instrument handle"=w146) -> ("error out"=w81:errorcluster, "actual points"=w70:i32, "amplitude"=w76:dbl[], "instrument handle out"=w127:refnum<k15>)  [unwired: 3 in]
          "tracedata" <- w76
          "actual points" <- w70
          n58 = flat-sequence {
            tunnel: w81 -> [w206]
            tunnel: [w206] -> w80
            tunnel: w79 -> [w205]
            tunnel: [w204] -> w73
            tunnel: w76 -> [w201]
            tunnel: w70 -> [w196]
            frame #0 {
              w202 = "\r\n"
              n59 = Number To Fractional String(number=w201, precision (6)=i16 2) -> (F-format string=w199:string[])  [unwired: 2 in]
              n60 = Array Subset(array=w199, length=w196) -> (w197:string[])  [unwired: 1 in]
              n61 = for {
                tunnel: w197 -> [w209] mode=indexing
                tunnel: [w207] -> w198 mode=indexing
                n62 = Concatenate Strings(w209, "\r\n") -> (w207:string)
              }
              n63 = Concatenate Strings(w205, w198, w202, "-------- DEMO POWER SUITE MEASUREMENT-------" ("y"), w202) -> (w204:string)
            }
          }
          n64 = local write "Display Details"(w73) -> ()
          n65 = Unbundle By Name("DEMO POWER SUITE MEASUREMENT") -> ("Scale"=w98:dbl, "Continuous MM"=w100:bool, "Input Amplitude Reference"=w101:i32, "Frequency Span"=w102:dbl, "Center Frequency"=w103:dbl)
          n66 = call <instrlib>:"SetAttributeViReal64.vi"("AttributeValue"=w103, "error in (no error)"=w80, "AttributeID"=w136, "RepCapIdentifier"=w141, "instrument handle"=w127) -> ("error out"=w131:errorcluster, "instrument handle out"=w135:refnum<k15>)  [unwired: 5 in]
          n67 = call <instrlib>:"SetAttributeViReal64.vi"("AttributeValue"=w102, "error in (no error)"=w131, "AttributeID"=w134, "RepCapIdentifier"=w141, "instrument handle"=w135) -> ("error out"=w132:errorcluster, "instrument handle out"=w133:refnum<k15>)  [unwired: 5 in]
          n68 = call <instrlib>:"SetAttributeViInt32.vi"("AttributeValue"=w101, "error in (no error)"=w132, "AttributeID"=w137, "RepCapIdentifier"=w141, "instrument handle"=w133) -> ("error out"=w129:errorcluster, "instrument handle out"=w130:refnum<k15>)  [unwired: 5 in]
          n69 = call <instrlib>:"SetAttributeViBoolean_Advanced.vi"("AttributeValue (Off)"=w100, "error in (no error)"=w129, "AttributeID"=w128, "RepCapIdentifier"=w141, "instrument handle"=w130) -> ("error out"=w139:errorcluster, "instrument handle out"=w138:refnum<k15>)  [unwired: 5 in]
          n70 = call <instrlib>:"SetAttributeViReal64.vi"("AttributeValue"=w98, "error in (no error)"=w139, "AttributeID"=w140, "RepCapIdentifier"=w141, "instrument handle"=w138) -> ("error out"=w78:errorcluster, "instrument handle out"=w126:refnum<k15>)  [unwired: 5 in]
          n71 = call <instrlib>:"SAPowerStatisticsTracesInitiate.vi"("error in (no error)"=w78, "instrument handle"=w126) -> ("error out"=w124:errorcluster, "instrument handle out"=w125:refnum<k15>)  [unwired: 8 in]
          n72 = call <instrlib>:"SAPowerStatisticsTraceRead.vi"("RetValBufferSize"="RetValBufferSize", "error in (no error)"=w124, "MaxTime"="MaxTime", "RepCapIdentifier"="RepCapIdentifier", "instrument handle"=w125) -> ("error out"=w123:errorcluster, "RetValActualSize"=w68:i32, "RetVal"=w74:dbl[], "instrument handle out"=w119:refnum<k15>)  [unwired: 3 in]
          "RetValActualSize" <- w68
          "RetVal" <- w74
          n73 = Number To Fractional String(number=w74, precision (6)=i16 2) -> (F-format string=w69:string[])  [unwired: 2 in]
          n74 = Array Subset(array=w69, length=w68) -> (w67:string[])  [unwired: 1 in]
          n75 = for {
            tunnel: w67 -> [w195] mode=indexing
            tunnel: [w193] -> w72 mode=indexing
            n76 = Concatenate Strings(w195, "\r\n") -> (w193:string)
          }
          n77 = Concatenate Strings(w73, w72) -> (w71:string)
        }
        frame True {
          n78 = Concatenate Strings(w241, "M9420A, M9421A, M90XA and M8920A doesn't supports the SA application, it only supports few basic SA common commands, so this example will not work fully with this model." ("y"), "\r\n") -> (w239:string)
        }
      }
    }
    frame Error {
    }
  }
  n79 = call <instrlib>:"Close.vi"("error in (no error)"=w8, "instrument handle"=w5) -> ("error out"=w1:errorcluster)  [unwired: 9 in]
  n80 = case shown="No Error" w1 {
    tunnel: w1 -> [w262 w268]
    tunnel: [w261 w268] -> w4
    tunnel: w3 -> [w260 w269]
    tunnel: [w259 w269] -> w2
    frame No Error {
      n81 = flat-sequence {
        tunnel: w262 -> [w267]
        tunnel: [w267] -> w261
        tunnel: w260 -> [w266]
        tunnel: [w265] -> w259
        frame #0 {
          n82 = Concatenate Strings(w266, "\r\n", "Driver Closed.") -> (w265:string)
        }
      }
    }
    frame Error {
    }
  }
  "Display Details" <- w2
  n83 = call <vilib>:"Simple Error Handler.vi"("error in (no error)"=w4) -> ()  [unwired: 4 in, 5 out]
